vi "Transfer file to roboRIO.vi"(8 "error in (no error)":errorcluster, 11 "Configuration File Path":path) -> (0 "error out":errorcluster, 3 "String":string)   [LabVIEW 2018]
doc: "This VI opens a system configuration request to query any roboRIO connected to the computer and sends the file to the first one that it finds."
uses:
  <vilib>/FTP/NI_FTP.lvlib
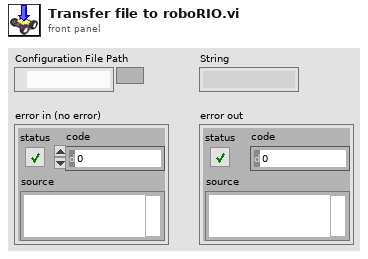
[diagram p1: front panel]
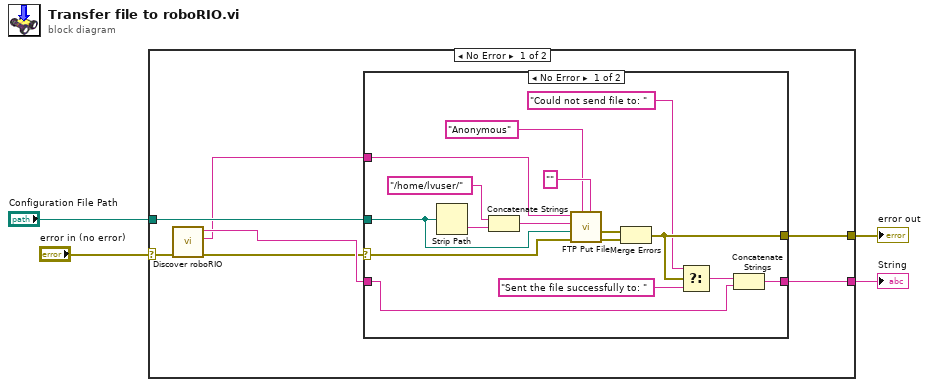
[diagram p0: block diagram]
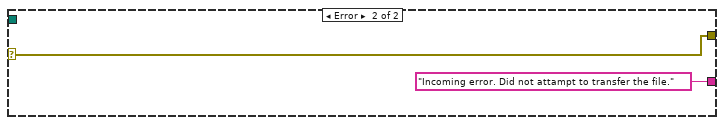
[diagram p3: hidden frame]
diagram:
  n1 = case shown="No Error" "error in (no error)" {
    selector: "error in (no error)" -> [w10 w31]
    tunnel: [w6 "Incoming error. Did not attampt to transfer the file."] -> w4
    tunnel: [w9 w31] -> w3
    tunnel: "Configuration File Path" -> [w11 _]
    frame No Error {
      n2 = call "Discover roboRIO.vi"("error in (no error)"=w10) -> ("error out"=w5:errorcluster, "roboRIO IP address"=w7:string, "roboRIO name"=w8:string)  [unwired: 8 in]
      n3 = case shown="No Error" w5 {
        selector: w5 -> [w12 w29]
        tunnel: w11 -> [w27 _]
        tunnel: [w25 w29] -> w9
        tunnel: w8 -> [w22 w28]
        tunnel: w7 -> [w16 _]
        tunnel: [w15 w28] -> w6
        frame No Error {
          n4 = Strip Path(path=w27) -> (name=w14:string)  [unwired: 1 out]
          n5 = Concatenate Strings("/home/lvuser/" ("remote path"), w14) -> (w13:string)
          n6 = call <vilib>:"FTP Put File.vi"("password"="", "user"="Anonymous", "error in (no error)"=w12, "local path"=w27, "remote path"=w13, "host"=w16) -> ("error out"=w24:errorcluster, "file error"=w23:errorcluster)  [unwired: 4 in]
          n7 = Merge Errors(w23, w24) -> (w25:errorcluster)
          n8 = Select(t="Could not send file to: " ("user"), s=w25, f="Sent the file successfully to: " ("user")) -> (s? t:f=w26:string)
          n9 = Concatenate Strings(w26, w22) -> (w15:string)
        }
        frame Error {
        }
      }
    }
    frame Error {
    }
  }
  "String" <- w4
  "error out" <- w3
